vi "Mass spectrometer.vi"() -> ()   [LabVIEW 2012]
doc: "Use this template to build a standard state machine design pattern. Each state executes code and determines which state to transition to. Contrast this design pattern with the User Interface Event Handler pattern, in which code executes in response to user actions. Contrast this design pattern also with the Queued Message Handler pattern, in which each message handling code can queue zero or more new messages.\nNote: This template does not contain the most recent programming guidelines recommended by National Instruments. For a complete, project-based implementation of the Standard State Machine pattern, use the Create Project dialog box instead of this template."
uses:
  SpektrometrMaszBibliot.ctl
panel:
  out "XY Graph":cluster{dbl[], dbl[]}(graph)
  in  "max Up":dbl=1000.0
  in  "min Up":dbl=600.0
  in  "zwiekszaj Up o":dbl=1.0
  in  "skan":bool
  in  "stop":bool
  out "U jon":dbl
  out "U przysp":dbl
  in  "Ie":dbl
  in  "Up":dbl
  in  "Zapis":refnum<visa-resource-name>="COM12"
  in  "Odczyt":refnum<visa-resource-name>="COM13"
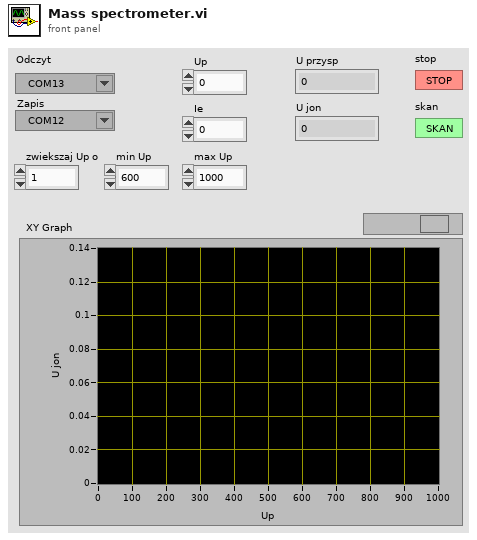
[diagram p1: front panel]
types:
  T1 = typedef "SpektrometrMaszBibliot.ctl" = enum16{"Initialize", "Zapisz", "Czytaj U prz", "Czytaj U jon", "Stop", "Skan"}
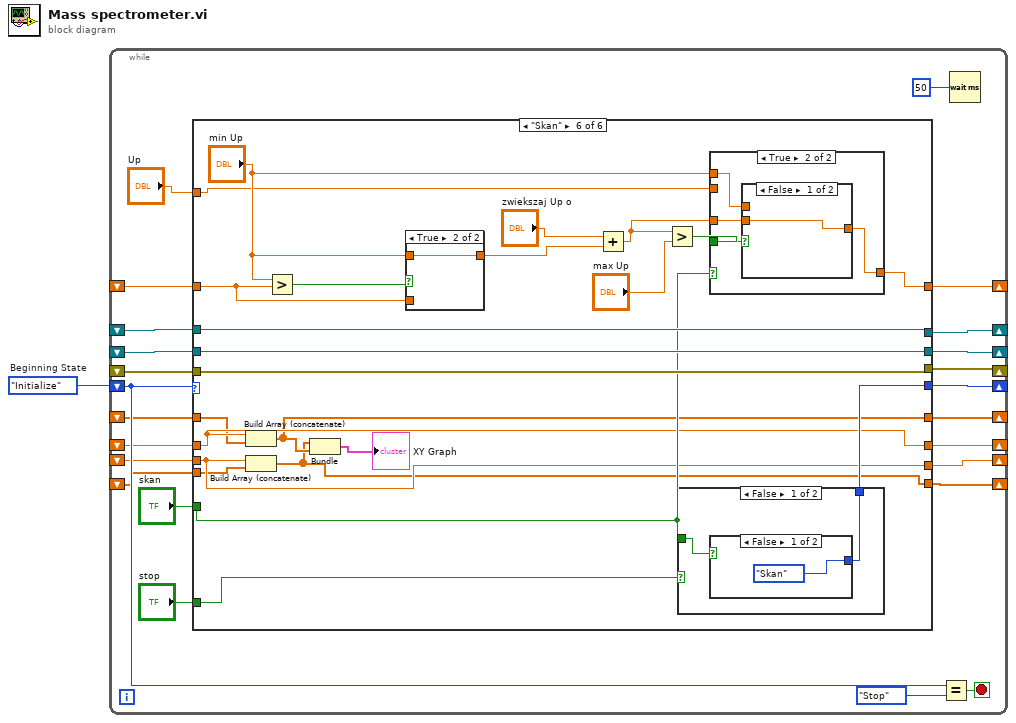
[diagram p0: block diagram]
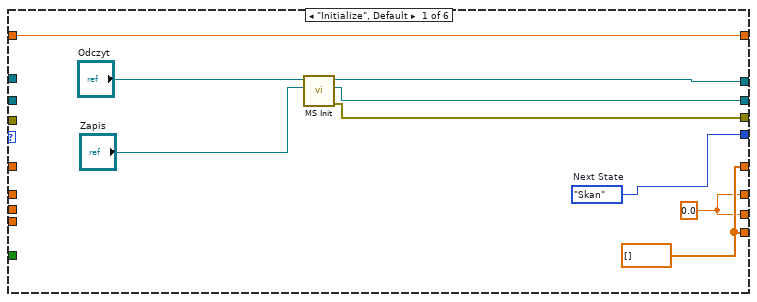
[diagram p2: hidden frame]
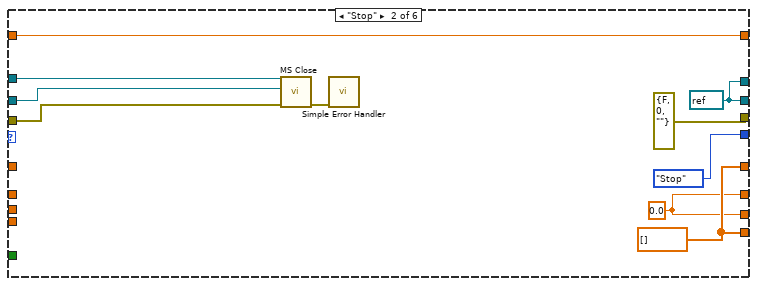
[diagram p3: hidden frame]
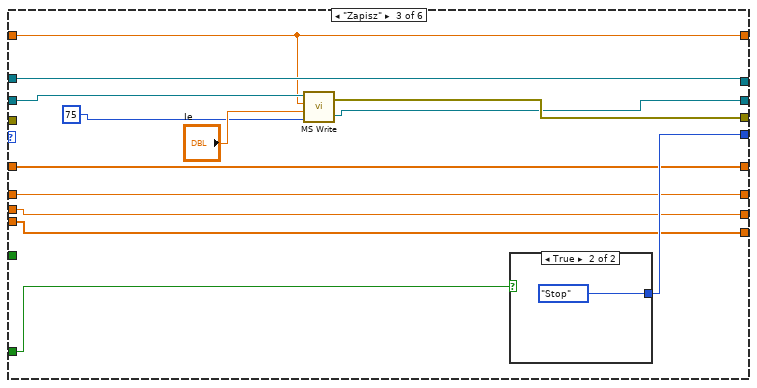
[diagram p4: hidden frame]
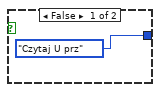
[diagram p5: hidden frame]
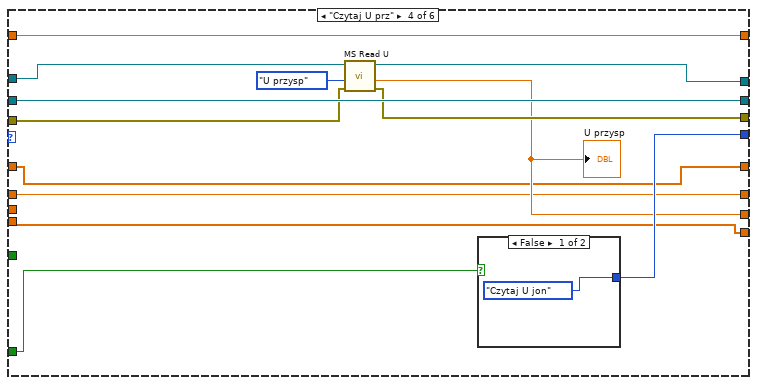
[diagram p6: hidden frame]
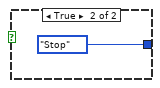
[diagram p7: hidden frame]
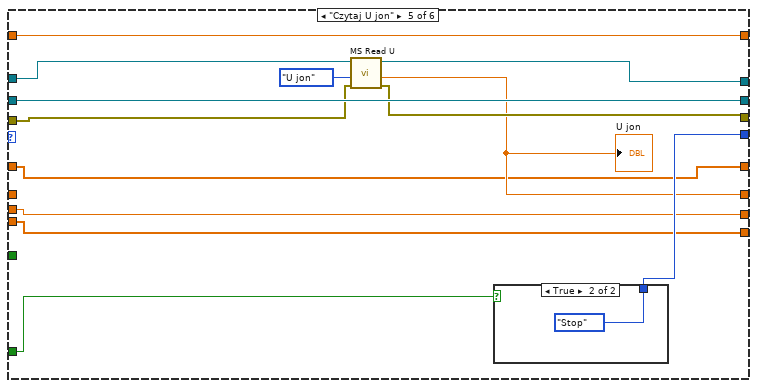
[diagram p8: hidden frame]
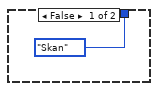
[diagram p9: hidden frame]
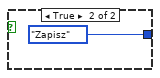
[diagram p13: hidden frame]
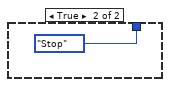
[diagram p14: hidden frame]
diagram:
  w1 = SpektrometrMaszBibliot."Initialize"  # Beginning State
  n1 = while {
    shift-right: [w22] -> _
    shift-left: w1 -> [w23]
    shift-right: [w19] -> _
    shift-left: _ -> [w17]
    shift-right: [w20] -> _
    shift-left: _ -> [w18]
    shift-right: [w16] -> _
    shift-left: _ -> [w15]
    shift-right: [w11] -> _
    shift-left: _ -> [w10]
    shift-right: [w8] -> _
    shift-left: _ -> [w7]
    shift-right: [w9] -> _
    shift-left: _ -> [w6]
    shift-right: [w5] -> _
    shift-left: _ -> [w3]
    shift-right: [w4] -> _
    shift-left: _ -> [w2]
    stop <- w25 stop-if-true
    n2 = case shown="\"Skan\"" w23 {
      tunnel: [w29 SpektrometrMaszBibliot."Stop" ("Next State") w51 w66 w81 w112] -> w22
      tunnel: [w32 w38 w56 w70 w83 w111] -> w20
      tunnel: [w31 w38 w54 w71 w85 w110] -> w19
      tunnel: w18 -> [_ w43 w56 w72 w86 w111]
      tunnel: w17 -> [_ w42 w57 w71 w85 w110]
      tunnel: [w30 errorcluster {"status"=FALSE, "code"=0, "source"=""} ("error out") w55 w69 w82 w109] -> w16
      tunnel: w15 -> [_ w41 _ w68 w84 w109]
      tunnel: "stop" -> [_ _ w52 w65 w80 w108]
      tunnel: "skan" -> [_ _ _ _ _ w98]
      tunnel: "Up" -> [_ _ _ _ _ w97]
      tunnel: [w28 w37 w49 w64 w79 w104] -> w11
      tunnel: w10 -> [w28 w37 w49 w64 w79 w99]
      tunnel: [w26 w35 w47 w63 w77 w96] -> w9
      tunnel: [w26 w35 w48 w62 w78 w95] -> w8
      tunnel: w7 -> [_ _ w48 w62 _ w95]
      tunnel: w6 -> [_ _ w47 _ w77 w96]
      tunnel: [w27 w36 w46 w61 w76 w92] -> w5
      tunnel: [w27 w36 w45 w60 w75 w91] -> w4
      tunnel: w3 -> [_ _ w46 w61 w76 w94]
      tunnel: w2 -> [_ _ w45 w60 w75 w93]
      frame "Initialize", Default {
        w26 = 0.0 ("Napiecie")
        w27 = dbl[] []
        w29 = SpektrometrMaszBibliot."Skan"  # Next State
        n3 = call "MS Init.vi"("VISA resource name"="Zapis", "VISA Refnum in"="Odczyt") -> ("error out"=w30:errorcluster, "VISA Refnum out 2"=w31:refnum<visa-resource-name>, "VISA Refnum out"=w32:refnum<visa-resource-name>)  [unwired: 7 in]
      }
      frame "Stop" {
        w35 = 0.0 ("Napiecie")
        w36 = dbl[] []
        w38 = refnum<visa-resource-name> refnum ("VISA Refnum out")
        n4 = call "MS Close.vi"("error in (no error)"=w41, "VISA Refnum in 2"=w42, "VISA Refnum in"=w43) -> ("error out"=w40:errorcluster)  [unwired: 8 in]
        n5 = call <vilib>:"Simple Error Handler.vi"("error in (no error)"=w40) -> ()  [unwired: 4 in, 5 out]
      }
      frame "Zapisz" {
        n6 = call "MS Write.vi"("VISA Refnum in"=w57, "Up"=w49, "Ie"="Ie", "delay"=u32 75) -> ("error out"=w55:errorcluster, "VISA Refnum out"=w54:refnum<visa-resource-name>)  [unwired: 1 in]
        n7 = case shown="True" w52 {
          tunnel: [SpektrometrMaszBibliot."Czytaj U prz" ("Next State") SpektrometrMaszBibliot."Stop" ("Next State")] -> w51
          frame False {
          }
          frame True {
          }
        }
      }
      frame "Czytaj U prz" {
        n8 = call "MS Read U.vi"("error in (no error)"=w68, "U (def. przysp)"=enum16{"U przysp", "U jon"}."U przysp", "VISA Refnum in"=w72) -> ("error out"=w69:errorcluster, "Napiecie"=w63:dbl, "VISA Refnum out"=w70:refnum<visa-resource-name>)  [unwired: 5 in, 1 out]
        "U przysp" <- w63
        n9 = case shown="False" w65 {
          tunnel: [SpektrometrMaszBibliot."Czytaj U jon" ("Next State") SpektrometrMaszBibliot."Stop" ("Next State")] -> w66
          frame False {
          }
          frame True {
          }
        }
      }
      frame "Czytaj U jon" {
        n10 = call "MS Read U.vi"("error in (no error)"=w84, "U (def. przysp)"=enum16{"U przysp", "U jon"}."U jon", "VISA Refnum in"=w86) -> ("error out"=w82:errorcluster, "Napiecie"=w78:dbl, "VISA Refnum out"=w83:refnum<visa-resource-name>)  [unwired: 5 in, 1 out]
        "U jon" <- w78
        n11 = case shown="True" w80 {
          tunnel: [SpektrometrMaszBibliot."Skan" ("Next State") SpektrometrMaszBibliot."Stop" ("Next State")] -> w81
          frame False {
          }
          frame True {
          }
        }
      }
      frame "Skan" {
        n12 = Build Array (concatenate)(w95, w94) -> (w92:dbl[])
        n13 = Build Array (concatenate)(w96, w93) -> (w91:dbl[])
        n14 = Greater?(x="min Up", y=w99) -> (0:w102:bool)
        n15 = Bundle(w91, w92) -> (→"XY Graph":cluster{dbl[], dbl[]})  [unwired: 1 in]
        n16 = case shown="True" w102 {
          tunnel: [w120 w121] -> w101
          tunnel: "min Up" -> [_ w121]
          tunnel: w99 -> [w120 _]
          frame False {
          }
          frame True {
          }
        }
        n17 = Add(x="zwiekszaj Up o", y=w101) -> (x+y=w103:dbl)
        n18 = Greater?(x=w103, y="max Up") -> (0:w105:bool)
        n19 = case shown="False" w108 {
          tunnel: [w123 SpektrometrMaszBibliot."Stop" ("Next State")] -> w112
          tunnel: w98 -> [w122 _]
          frame False {
            n20 = case shown="False" w122 {
              tunnel: [SpektrometrMaszBibliot."Skan" ("Next State") SpektrometrMaszBibliot."Zapisz" ("Next State")] -> w123
              frame False {
              }
              frame True {
              }
            }
          }
          frame True {
          }
        }
        n21 = case shown="True" w98 {
          tunnel: w105 -> [_ w117]
          tunnel: [w113 w116] -> w104
          tunnel: w103 -> [_ w115]
          tunnel: "min Up" -> [_ w114]
          tunnel: w97 -> [w113 _]
          frame False {
          }
          frame True {
            n22 = case shown="False" w117 {
              tunnel: [w118 w119] -> w116
              tunnel: w114 -> [_ w119]
              tunnel: w115 -> [w118 _]
              frame False {
              }
              frame True {
              }
            }
          }
        }
      }
    }
    n23 = Equal?(x=w23, y=SpektrometrMaszBibliot."Stop" ("States")) -> (x = y?=w25:bool)
    n24 = Wait (ms)(milliseconds to wait=u32 50) -> ()  [unwired: 1 out]
  }
